vi "Load Enabled Instruments.vi"(8 "error in (no error)":errorcluster, 11 "ManualUI in":refnum<class "ManualUI.lvclass">) -> (0 "error out":errorcluster, 3 "ManualUI out":refnum<class "ManualUI.lvclass">)   [LabVIEW 2023, in "ManualUI.lvlib" / "ManualUI.lvclass"]
uses:
  Library/ManualUI.lvclass
  Library/ManualUI.lvclass/ManualUI.ctl
  builds/Framework/Configuration.lvlibp/Library/Configuration.lvclass
  builds/Framework/Engine.lvlibp/Engine/Library/Engine.lvclass
  C:/Users/Public/Documents/Development/builds/Main/Docking.lvlibp/Prime Panel/PrimeDock.lvclass
  C:/Users/Public/Documents/Development/builds/Main/Docking.lvlibp/Docking/Docking.lvclass
  C:/Users/Public/Documents/Development/builds/Framework/Engine.lvlibp/Managed Actor/Library/Managed Actor.lvclass
  C:/Users/Public/Documents/Development/builds/Framework/Engine.lvlibp/Engine/Library/Engine.lvclass
  C:/Users/Public/Documents/Development/builds/Framework/Panel Manager.lvlibp/Library/Panel Actor.lvclass
  C:/Users/Public/Documents/Development/builds/Framework/Monitored Actor.lvlibp/Actor Monitor/Actor Monitor/Actor Monitor.lvclass
  C:/Users/Public/Documents/Development/builds/Framework/Actor Framework.lvlibp/1abvi3w/vi.lib/ActorFramework/Actor/Actor.lvclass
  C:/Users/Public/Documents/Development/Application/Prime Panels/ManualUI/Library/ManualUI.lvclass
  C:/Users/Public/Documents/Development/builds/Framework/Configuration.lvlibp/Library/Configuration.lvclass
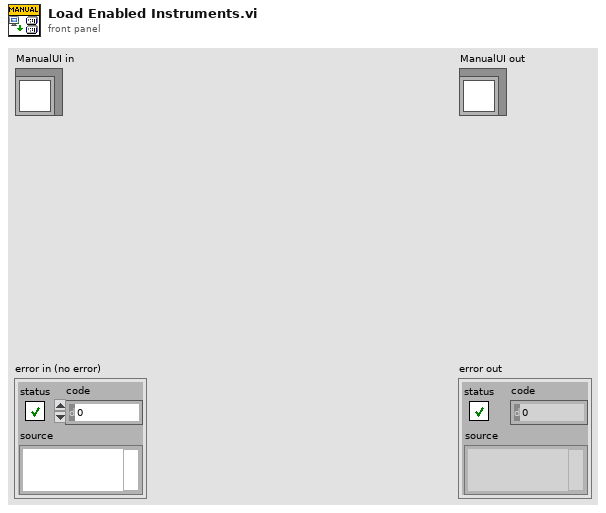
[diagram p1: front panel]
types:
  T1 = cluster{"String":string, "Instrument out":refnum<class "Instruments.lvclass">, i32}
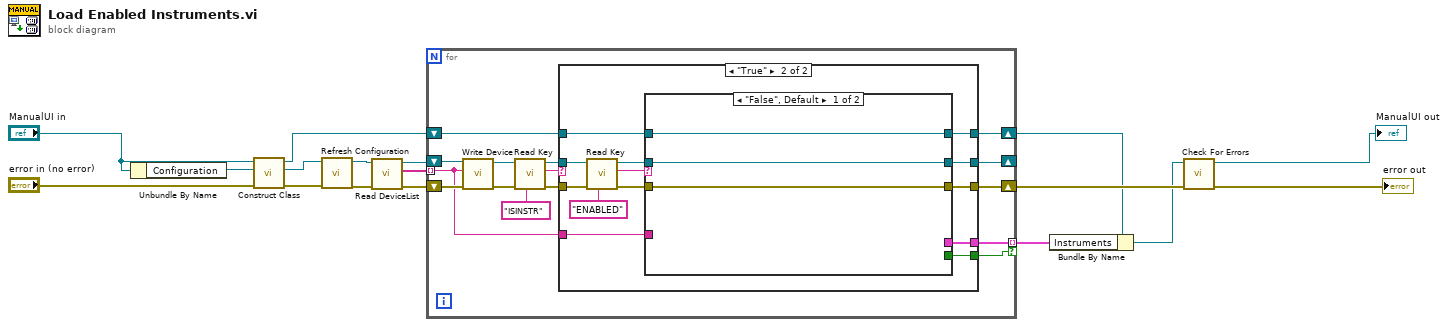
[diagram p0: block diagram]
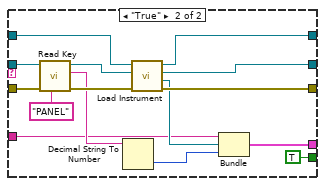
[diagram p3: hidden frame]
diagram:
  n1 = Unbundle By Name("ManualUI in") -> ("Configuration"=w16:refnum<class "Configuration.lvclass">)
  n2 = call "Construct Class.vi"("error in (no error)"="error in (no error)", "Actor in"=w16, "Engine in"="ManualUI in") -> ("error out"=w14:errorcluster, "Actor out"=w15:refnum<class "Configuration.lvclass">, "Engine out"=w13:refnum<class "ManualUI.lvclass">)  [unwired: 6 in]
  n3 = call "Refresh Configuration.vi"("error in (no error)"=w14, "Configuration in"=w15) -> ("error out"=w11:errorcluster, "Configuration out"=w12:refnum<class "Configuration.lvclass">)  [unwired: 8 in]
  n4 = call "Read DeviceList.vi"("error in (no error)"=w11, "Configuration in"=w12) -> ("error out"=w10:errorcluster, "DeviceList"=w8:string[], "Configuration out"=w9:refnum<class "Configuration.lvclass">)  [unwired: 7 in]
  n5 = for {
    shift-right: [w24] -> w6
    shift-left: w10 -> [w23]
    shift-right: [w21] -> w5
    shift-left: w13 -> [w22]
    tunnel: w8 -> [w20] mode=indexing
    shift-right: [w26] -> _
    shift-left: w9 -> [w32]
    tunnel: [w19] -> w4 mode=indexing if=w18
    n6 = call "Write Device.vi"("error in (no error)"=w23, "Device"=w20, "Configuration in"=w32) -> ("error out"=w30:errorcluster, "Configuration out"=w31:refnum<class "Configuration.lvclass">)  [unwired: 7 in]
    n7 = call "Read Key.vi"("Key"="ISINSTR", "error in (no error)"=w30, "Configuration in"=w31) -> ("error out"=w25:errorcluster, "Value"=w28:string, "Configuration out"=w27:refnum<class "Configuration.lvclass">)  [unwired: 6 in]
    n8 = case shown="\"True\"" w28 {
      tunnel: w27 -> [w35 w46]
      tunnel: [w35 w43] -> w26
      tunnel: w25 -> [w34 w47]
      tunnel: [w34 w41] -> w24
      tunnel: w22 -> [w33 w40]
      tunnel: [w33 w39] -> w21
      tunnel: w20 -> [_ w38]
      tunnel: [_ w37] -> w19
      tunnel: [_ w36] -> w18
      frame "False", Default {
      }
      frame "True" {
        n9 = call "Read Key.vi"("Key"="ENABLED", "error in (no error)"=w47, "Configuration in"=w46) -> ("error out"=w42:errorcluster, "Value"=w45:string, "Configuration out"=w44:refnum<class "Configuration.lvclass">)  [unwired: 6 in]
        n10 = case shown="\"False\", Default" w45 {
          tunnel: w44 -> [w51 w64]
          tunnel: [w51 w59] -> w43
          tunnel: w42 -> [w50 w65]
          tunnel: [w50 w58] -> w41
          tunnel: w40 -> [w49 w63]
          tunnel: [w49 w62] -> w39
          tunnel: w38 -> [_ w54]
          tunnel: [_ w53] -> w37
          tunnel: [_ TRUE] -> w36
          frame "False", Default {
          }
          frame "True" {
            n11 = call "Read Key.vi"("Key"="PANEL", "error in (no error)"=w65, "Configuration in"=w64) -> ("error out"=w60:errorcluster, "Value"=w56:string, "Configuration out"=w61:refnum<class "Configuration.lvclass">)  [unwired: 6 in]
            n12 = Decimal String To Number(string=w56) -> (number=w55:i32)  [unwired: 2 in, 1 out]
            n13 = call "Load Instrument.vi"("error in (no error)"=w60, "Configuration in"=w61, "ManualUI in"=w63) -> ("error out"=w58:errorcluster, "Instrument out"=w57:refnum<class "Instruments.lvclass">, "Configuration out"=w59:refnum<class "Configuration.lvclass">, "ManualUI out"=w62:refnum<class "ManualUI.lvclass">)  [unwired: 5 in]
            n14 = Bundle("String"=w54, "Instrument out"=w57, w55) -> (w53:T1)  [unwired: 1 in]
          }
        }
      }
    }
  }
  n15 = Bundle By Name(cluster=w5, "Instruments"=w4) -> (w2:refnum<class "ManualUI.lvclass">)
  n16 = call "Check For Errors.vi"("error in"=w6, "Engine in"=w2) -> ("error out"=→"error out":errorcluster, "Engine out"=→"ManualUI out":refnum<class "ManualUI.lvclass">)  [unwired: 8 in]
